vi "Set_Reset_AdmainX.vi"(2 "error in":errorcluster, 3 "device name":tag="Dev0", 4 "ADMAINX":u8) -> (0 "error out":errorcluster)   [LabVIEW 2017]
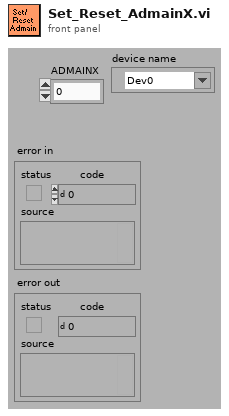
[diagram p1: front panel]
types:
  T1 = enum16{"Reset", "Update U1", "Update U2", "Update U3", "Read all"}
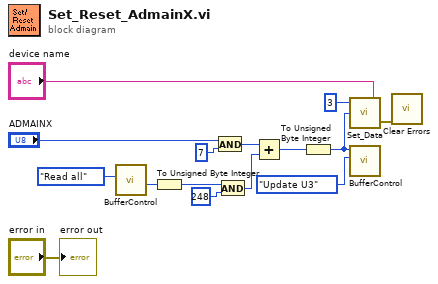
[diagram p0: block diagram]
diagram:
  n1 = call "BufferControl.vi"("Enum"=T1."Read all") -> ("U3BuffRead"=w3:u8)  [unwired: 3 in, 3 out]
  n2 = To Unsigned Byte Integer(number=w3) -> (unsigned 8bit integer=w7:u8)
  n3 = And(x="ADMAINX", y=u16 7) -> (x .and. y?=w6:u16)
  n4 = And(x=w7, y=u16 248) -> (x .and. y?=w5:u16)
  n5 = Add(x=w6, y=w5) -> (x+y=w4:u16)
  n6 = To Unsigned Byte Integer(number=w4) -> (unsigned 8bit integer=w12:u8)
  n7 = call "Set_Data.vi"("device name"="device name", "Data"=w12, "Ch"=u8 3) -> ("error out"=w1:errorcluster)  [unwired: 1 in]
  n8 = call "BufferControl.vi"("Enum"=T1."Update U3", "Data"=w12) -> ()  [unwired: 2 in, 4 out]
  n9 = call <vilib>:"Clear Errors.vi"("error in (no error)"=w1) -> ()  [unwired: 5 in, 2 out]
  "error out" <- "error in"
